vi "repair-tags.vi"() -> ()   [LabVIEW 2013]
uses:
  tags_cluster.ctl
  imagereconstruction/x64/Release/labviewdll.dll
panel:
  in  "Fix page numbers":bool
  out "String":string
  out "Inital Properties":T1
  in  "Path":path
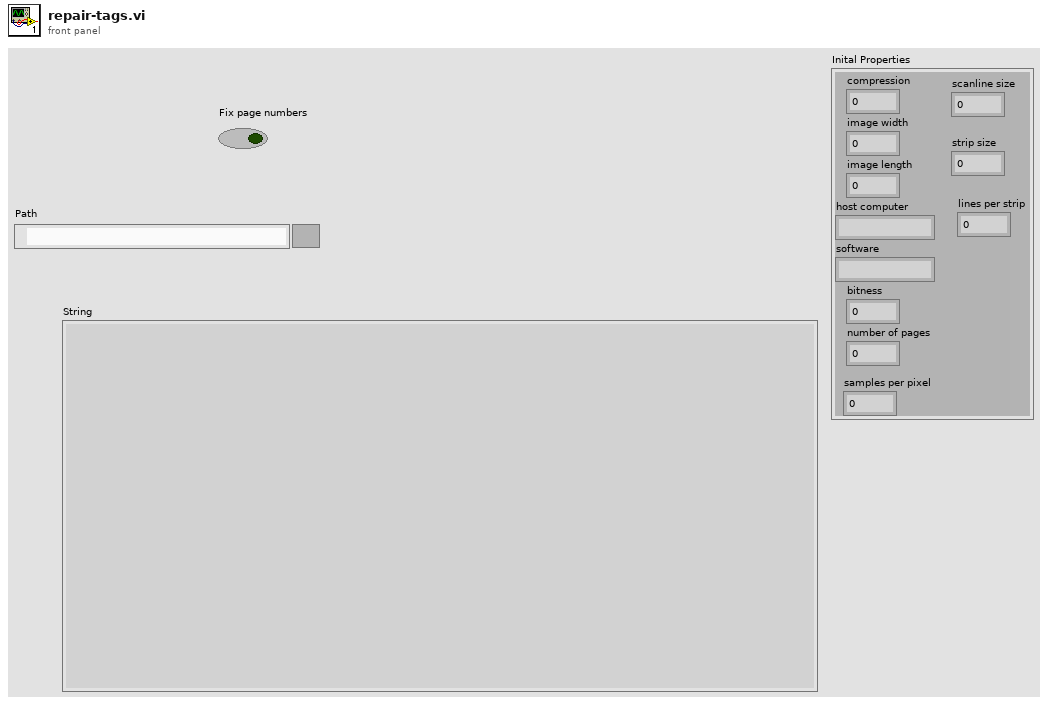
[diagram p1: front panel]
types:
  T1 = typedef "tags_cluster.ctl" = cluster{"compression":i32, "image width":i32, "image length":i32, "host computer":string, "software":string, "bitness":i32, "number of pages":i32, "samples per pixel":i32, "scanline size":i32, "strip size":i32, "lines per strip":i32}
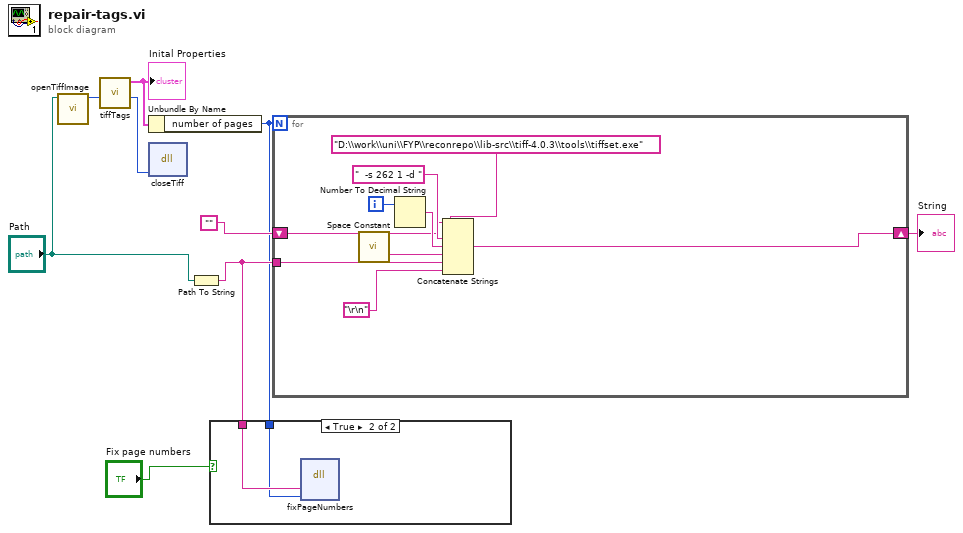
[diagram p0: block diagram]
diagram:
  n1 = call "openTiffImage.vi"("Path string"="Path") -> ("returned pointer"=w9:i64)  [unwired: 9 in, 1 out]
  n2 = call "tiffTags.vi"("tif pointer"=w9) -> ("tiff pointer"=w7:i64, "Image Properties"=w8:T1)  [unwired: 8 in, 1 out]
  "Inital Properties" <- w8
  n3 = Unbundle By Name(w8) -> ("number of pages"=w1:i32)
  n4 = dll-call lib="D:/work/uni/FYP/reconrepo/imagereconstruction/x64/Debug/labviewdll.dll" fn="closeTiff"("tiff"=w7) -> ()  [unwired: 5 in, 2 out]
  n5 = Path To String(path="Path") -> (string=w2:string)
  n6 = case shown="True" "Fix page numbers" {
    tunnel: w2 -> [_ w11]
    tunnel: w1 -> [_ w10]
    frame False {
    }
    frame True {
      n7 = dll-call lib="D:/work/uni/FYP/reconrepo/imagereconstruction/x64/Release/labviewdll.dll" fn="fixPageNumbers"("pathName"=w11, "npages"=w10) -> ()  [unwired: 6 in, 2 out]
    }
  }
  n8 = for {
    N: w1 -> [_]
    tunnel: w2 -> [w16]
    shift-right: [w12] -> w4
    shift-left: "" -> [w14]
    i -> [w19]
    n9 = call <vilib>:"Space Constant.vi"() -> ("String"=w17:string)
    n10 = Number To Decimal String(number=w19) -> (decimal integer string=w18:string)  [unwired: 1 in]
    n11 = Concatenate Strings(w14, "D:\\work\\uni\\FYP\\reconrepo\\lib-src\\tiff-4.0.3\\tools\\tiffset.exe" ("string"), "  -s 262 1 -d " ("string"), w18, w17, w16, "\r\n") -> (w12:string)
  }
  "String" <- w4
